vi "subVI_SimpleVolt.vi"() -> ()   [LabVIEW 2013]
uses:
  <vilib>/Utility/error.llb/DialogType.ctl
  <vilib>/DAQmx/read.llb/DAQmx Read (Analog 1D Wfm NChan NSamp).vi
  <vilib>/DAQmx/create/channels.llb/DAQmx Create Channel (AI-Voltage-Basic).vi
  <vilib>/DAQmx/configure/timing.llb/DAQmx Timing (Sample Clock).vi
  <vilib>/DAQmx/miscellaneous.llb/DAQmx Fill In Error Info.vi
  <resource>/objmgr/daqmx.rc
panel:
  out "숫자형":i32
  in  "정지":bool
  out "웨이브폼 그래프 2":waveform(dbl)[](graph)
  out "웨이브폼 그래프":waveform(dbl)[](graph)
  in  "샘플 개수":i32=100
  in  "샘플 속도":dbl=1000.0
  in  "샘플 클럭 소스":tag="OnboardClock"
  in  "터미널 설정":i32(ring)=-1 items=["기본값"=-1, "RSE"=10083, "NRSE"=10078, "차동"=10106, "유사 차동"=12529]
  in  "최대 전압":dbl=5.0
  in  "최소 전압":dbl=-5.0
  in  "물리적인 채널":tag="Dev1/ai0"
  out "실제 샘플 속도":dbl=1000.0 format="%0.2f"
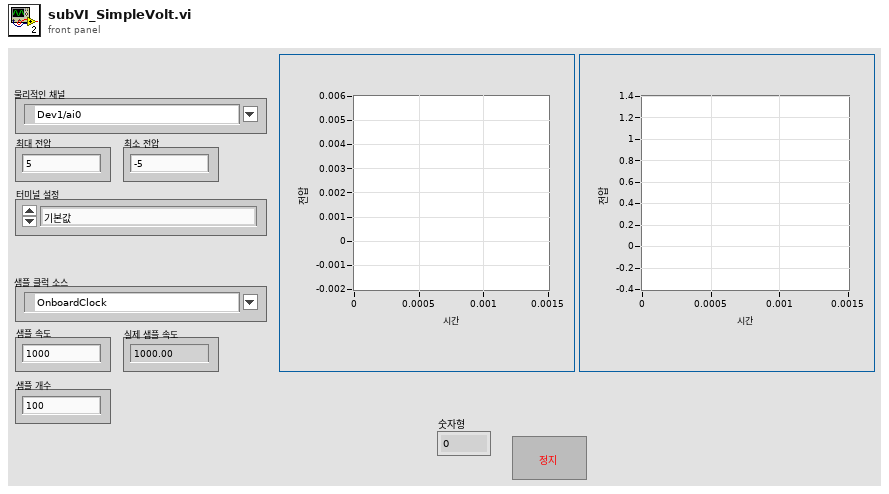
[diagram p1: front panel]
types:
  T1 = typedef "DialogType.ctl" = u16
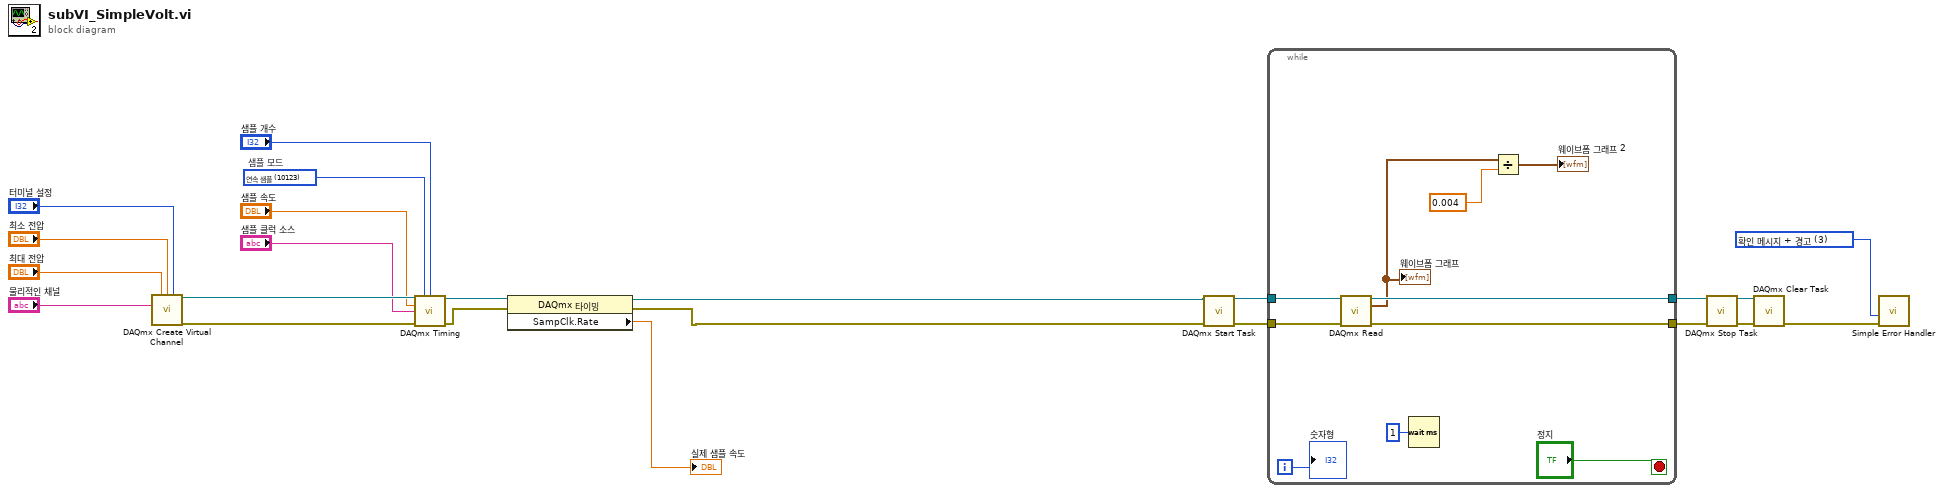
[diagram p0: block diagram]
diagram:
  w3 = T1 3 items=["대화 상자 없음", "확인 메시지", "메시지 지속 또는 정지", "확인 메시지 + 경고", "지속/정지 + 경고"] ("대화 상자 타입 (확인 메시지:1)")
  w21 = 10123 items=["유한 샘플"=10178, "연속 샘플"=10123, "하드웨어 타이밍에 의한 단일 포인트"=12522]  # 샘플 모드
  n1 = call-poly <vilib>:"DAQmx Create Virtual Channel.vi"("maximum value"="최대 전압", "minimum value"="최소 전압", "input terminal configuration"="터미널 설정", "physical channels"="물리적인 채널") -> ("task out"=w19:refnum<k21>, "error out"=w20:errorcluster)  [unwired: 10 in]
  n2 = call-poly <vilib>:"DAQmx Timing.vi"("task/channels in"=w19, "sample mode"=w21, "samples per channel"="샘플 개수", "rate"="샘플 속도", "source"="샘플 클럭 소스", "error in"=w20) -> ("task out"=w23:refnum<k21>, "error out"=w22:errorcluster)  [unwired: 8 in]
  n3 = property class="DAQmx 타이밍"(reference=w23, error in=w22) -> (reference out=w1:refnum<k21>, error out=w2:errorcluster, "SampClk.Rate"=→"실제 샘플 속도":dbl)
  n4 = call <vilib>:"DAQmx Start Task.vi"("task/channels in"=w1, "error in"=w2) -> ("task out"=w18:refnum<k21>, "error out"=w17:errorcluster)  [unwired: 12 in]
  n5 = while {
    tunnel: w18 -> [w33]
    tunnel: w17 -> [w32]
    tunnel: [w31] -> w5
    tunnel: [w30] -> w4
    i -> [w24]
    stop <- "정지" stop-if-true
    n6 = call-poly <vilib>:"DAQmx Read.vi"("task/channels in"=w33, "error in"=w32) -> ("task out"=w31:refnum<k21>, "data"=w28:waveform(dbl)[], "error out"=w30:errorcluster)  [unwired: 11 in]
    "웨이브폼 그래프" <- w28
    n7 = Wait (ms)(milliseconds to wait=u32 1 ("대기 시간(ms)")) -> ()  [unwired: 1 out]
    n8 = Divide(x=w28, y=0.004) -> (x/y=→"웨이브폼 그래프 2":waveform(dbl)[])
    "숫자형" <- w24
  }
  n9 = call <vilib>:"DAQmx Stop Task.vi"("task/channels in"=w5, "error in"=w4) -> ("task out"=w7:refnum<k21>, "error out"=w6:errorcluster)  [unwired: 12 in]
  n10 = call <vilib>:"DAQmx Clear Task.vi"("task in"=w7, "error in"=w6) -> ("error out"=w16:errorcluster)  [unwired: 13 in]
  n11 = call <vilib>:"Simple Error Handler.vi"("type of dialog (OK msg:1)"=w3, "error in (no error)"=w16) -> ()  [unwired: 3 in, 5 out]
